vi "AO Create.vi"(8 "error in (no error)":errorcluster, 10 "Analog_Configuration_Parameters":T1, 11 "C100L in":refnum<class "C100L.lvclass">) -> (0 "error out":errorcluster, 3 "C100L out":refnum<class "C100L.lvclass">)   [LabVIEW 2021, in "C100L.lvlib" / "C100L.lvclass"]
uses:
  C100L.lvclass
  <vilib>/NathanCo/Analog-Tasks/Utilities/Analog Configuration Parameters.ctl
  C100L.lvclass/C100L.ctl
  <vilib>/NathanCo/Analog-Tasks/Analog Output/Analog Output/Analog Output.lvclass
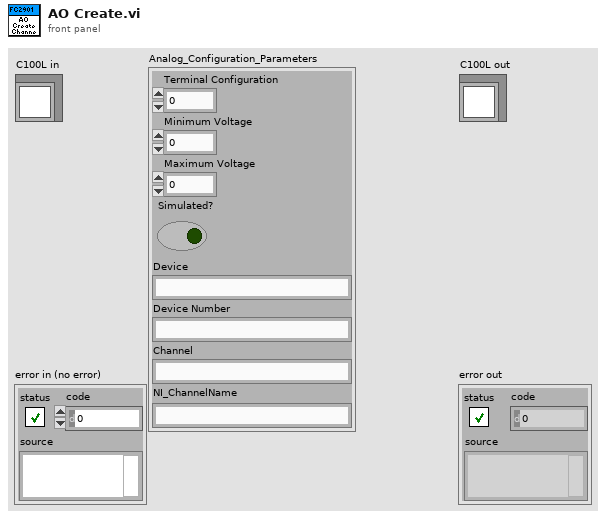
[diagram p1: front panel]
types:
  T1 = typedef "Analog Configuration Parameters.ctl" = cluster{"Terminal Configuration":i32, "Minimum Voltage":dbl, "Maximum Voltage":dbl, "Simulated?":bool, "Device":string, "Device Number":string, "Channel":string, "NI_ChannelName":string}
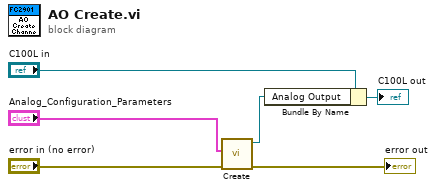
[diagram p0: block diagram]
diagram:
  n1 = call <vilib>:"Create.vi"("error in (no error)"="error in (no error)", "Analog_Configuration_Parameters"="Analog_Configuration_Parameters") -> ("error out"=→"error out":errorcluster, "Analog Output out"=w3:refnum<class "Analog Output.lvclass">)  [unwired: 8 in]
  n2 = Bundle By Name(cluster="C100L in", "Analog Output"=w3) -> (→"C100L out":refnum<class "C100L.lvclass">)
